vi "DataIn.vi"(2 "DeviceHandle":i32, 3 "SampleNumber":i32=1024) -> (0 "Error":bool, 1 "DataBuffer":u16[](array[numeric]))   [LabVIEW 2012]
uses:
  MPS-060602.dll
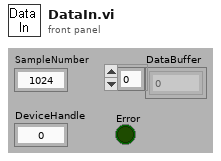
[diagram p1: front panel]
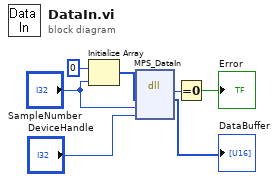
[diagram p0: block diagram]
diagram:
  n1 = Initialize Array(u16 0 ("element"), "SampleNumber") -> (w3:u16[])
  n2 = dll-call lib="PTH1Yabs CDocuments and Settings\nAdministrator桌面性能\tdriver VIMPS-060602.dll" fn="MPS_DataIn"("DataArray"=w3, "SampleNumber"="SampleNumber", "DeviceHandle"="DeviceHandle") -> (w7:i32, "DataArray"=→"DataBuffer":u16[])  [unwired: 5 in, 2 out]
  n3 = Equal To 0?(x=w7) -> (x = 0?=→"Error":bool)
